vi "9229_SampleRates.vi"(9 "error in (no error)":errorcluster, 11 "Data Rate [S/s]":u32) -> (1 "error out":errorcluster, 3 "Data Rate":T1=4 items=["51.200 kS/s (NI 9229)"=1, "25.600 kS/s (NI 9229)"=2, "17.067 kS/s (NI 9229)"=3, "12.800 kS/s (NI 9229)"=4, "10.240 kS/s (NI 9229)"=5, "8.533 kS/s (NI 9229)"=6, "7.314 kS/s (NI 9229)"=7, "6.400 kS/s (NI 9229)"=8, "5.689 kS/s (NI 9229)"=9, "5.120 kS/s (NI 9229)"=10, "4.654 kS/s (NI 9229)"=11, "4.267 kS/s (NI 9229)"=12, "3.938 kS/s (NI 9229)"=13, "3.657 kS/s (NI 9229)"=14, "3.413 kS/s (NI 9229)"=15, "3.200 kS/s (NI 9229)"=16, "3.012 kS/s (NI 9229)"=17, "2.845 kS/s (NI 9229)"=18, "2.695 kS/s (NI 9229)"=19, "2.560 kS/s (NI 9229)"=20, "2.438 kS/s (NI 9229)"=21, "2.328 kS/s (NI 9229)"=22, "2.226 kS/s (NI 9229)"=23, "2.133 kS/s (NI 9229)"=24, "2.048 kS/s (NI 9229)"=25, "1.969 kS/s (NI 9229)"=26, "1.896 kS/s (NI 9229)"=27, "1.829 kS/s (NI 9229)"=28, "1.765 kS/s (NI 9229)"=29, "1.707 kS/s (NI 9229)"=30, "1.652 kS/s (NI 9229)"=31])   [LabVIEW 2017]
uses:
  <vilib>/LabVIEW Targets/FPGA/cRIO/shared/nicrio_ModuleControls/nicrio_cRIO-9229_DataRatesRing2.ctl
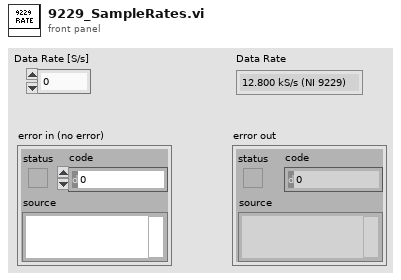
[diagram p1: front panel]
types:
  T1 = typedef "nicrio_cRIO-9229_DataRatesRing2.ctl" = u8
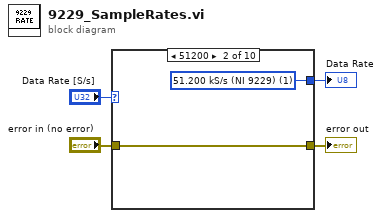
[diagram p0: block diagram]
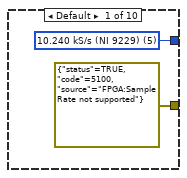
[diagram p2: hidden frame]
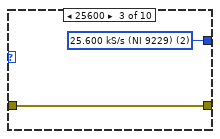
[diagram p3: hidden frame]
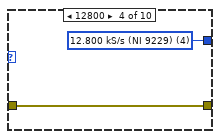
[diagram p4: hidden frame]
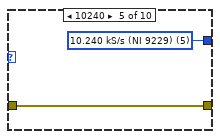
[diagram p5: hidden frame]
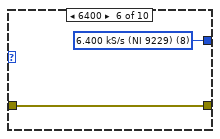
[diagram p6: hidden frame]
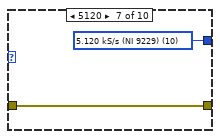
[diagram p7: hidden frame]
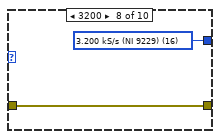
[diagram p8: hidden frame]
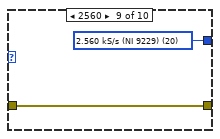
[diagram p9: hidden frame]
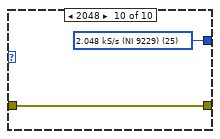
[diagram p10: hidden frame]
diagram:
  n1 = case shown="51200" "Data Rate [S/s]" {
    tunnel: [w5 w7 w9 w11 w13 w15 w17 w19 w21 w23] -> w3
    tunnel: "error in (no error)" -> [_ w8 w10 w12 w14 w16 w18 w20 w22 w24]
    tunnel: [errorcluster {"status"=TRUE, "code"=5100, "source"="FPGA:Sample Rate not supported"} ("error IO") w8 w10 w12 w14 w16 w18 w20 w22 w24] -> w1
    frame Default {
      w5 = T1 5 items=["51.200 kS/s (NI 9229)"=1, "25.600 kS/s (NI 9229)"=2, "17.067 kS/s (NI 9229)"=3, "12.800 kS/s (NI 9229)"=4, "10.240 kS/s (NI 9229)"=5, "8.533 kS/s (NI 9229)"=6, "7.314 kS/s (NI 9229)"=7, "6.400 kS/s (NI 9229)"=8, "5.689 kS/s (NI 9229)"=9, "5.120 kS/s (NI 9229)"=10, "4.654 kS/s (NI 9229)"=11, "4.267 kS/s (NI 9229)"=12, "3.938 kS/s (NI 9229)"=13, "3.657 kS/s (NI 9229)"=14, "3.413 kS/s (NI 9229)"=15, "3.200 kS/s (NI 9229)"=16, "3.012 kS/s (NI 9229)"=17, "2.845 kS/s (NI 9229)"=18, "2.695 kS/s (NI 9229)"=19, "2.560 kS/s (NI 9229)"=20, "2.438 kS/s (NI 9229)"=21, "2.328 kS/s (NI 9229)"=22, "2.226 kS/s (NI 9229)"=23, "2.133 kS/s (NI 9229)"=24, "2.048 kS/s (NI 9229)"=25, "1.969 kS/s (NI 9229)"=26, "1.896 kS/s (NI 9229)"=27, "1.829 kS/s (NI 9229)"=28, "1.765 kS/s (NI 9229)"=29, "1.707 kS/s (NI 9229)"=30, "1.652 kS/s (NI 9229)"=31] ("Data Rate")
    }
    frame 51200 {
      w7 = T1 1 items=["51.200 kS/s (NI 9229)"=1, "25.600 kS/s (NI 9229)"=2, "17.067 kS/s (NI 9229)"=3, "12.800 kS/s (NI 9229)"=4, "10.240 kS/s (NI 9229)"=5, "8.533 kS/s (NI 9229)"=6, "7.314 kS/s (NI 9229)"=7, "6.400 kS/s (NI 9229)"=8, "5.689 kS/s (NI 9229)"=9, "5.120 kS/s (NI 9229)"=10, "4.654 kS/s (NI 9229)"=11, "4.267 kS/s (NI 9229)"=12, "3.938 kS/s (NI 9229)"=13, "3.657 kS/s (NI 9229)"=14, "3.413 kS/s (NI 9229)"=15, "3.200 kS/s (NI 9229)"=16, "3.012 kS/s (NI 9229)"=17, "2.845 kS/s (NI 9229)"=18, "2.695 kS/s (NI 9229)"=19, "2.560 kS/s (NI 9229)"=20, "2.438 kS/s (NI 9229)"=21, "2.328 kS/s (NI 9229)"=22, "2.226 kS/s (NI 9229)"=23, "2.133 kS/s (NI 9229)"=24, "2.048 kS/s (NI 9229)"=25, "1.969 kS/s (NI 9229)"=26, "1.896 kS/s (NI 9229)"=27, "1.829 kS/s (NI 9229)"=28, "1.765 kS/s (NI 9229)"=29, "1.707 kS/s (NI 9229)"=30, "1.652 kS/s (NI 9229)"=31] ("Data Rate")
    }
    frame 25600 {
      w9 = T1 2 items=["51.200 kS/s (NI 9229)"=1, "25.600 kS/s (NI 9229)"=2, "17.067 kS/s (NI 9229)"=3, "12.800 kS/s (NI 9229)"=4, "10.240 kS/s (NI 9229)"=5, "8.533 kS/s (NI 9229)"=6, "7.314 kS/s (NI 9229)"=7, "6.400 kS/s (NI 9229)"=8, "5.689 kS/s (NI 9229)"=9, "5.120 kS/s (NI 9229)"=10, "4.654 kS/s (NI 9229)"=11, "4.267 kS/s (NI 9229)"=12, "3.938 kS/s (NI 9229)"=13, "3.657 kS/s (NI 9229)"=14, "3.413 kS/s (NI 9229)"=15, "3.200 kS/s (NI 9229)"=16, "3.012 kS/s (NI 9229)"=17, "2.845 kS/s (NI 9229)"=18, "2.695 kS/s (NI 9229)"=19, "2.560 kS/s (NI 9229)"=20, "2.438 kS/s (NI 9229)"=21, "2.328 kS/s (NI 9229)"=22, "2.226 kS/s (NI 9229)"=23, "2.133 kS/s (NI 9229)"=24, "2.048 kS/s (NI 9229)"=25, "1.969 kS/s (NI 9229)"=26, "1.896 kS/s (NI 9229)"=27, "1.829 kS/s (NI 9229)"=28, "1.765 kS/s (NI 9229)"=29, "1.707 kS/s (NI 9229)"=30, "1.652 kS/s (NI 9229)"=31] ("Data Rate")
    }
    frame 12800 {
      w11 = T1 4 items=["51.200 kS/s (NI 9229)"=1, "25.600 kS/s (NI 9229)"=2, "17.067 kS/s (NI 9229)"=3, "12.800 kS/s (NI 9229)"=4, "10.240 kS/s (NI 9229)"=5, "8.533 kS/s (NI 9229)"=6, "7.314 kS/s (NI 9229)"=7, "6.400 kS/s (NI 9229)"=8, "5.689 kS/s (NI 9229)"=9, "5.120 kS/s (NI 9229)"=10, "4.654 kS/s (NI 9229)"=11, "4.267 kS/s (NI 9229)"=12, "3.938 kS/s (NI 9229)"=13, "3.657 kS/s (NI 9229)"=14, "3.413 kS/s (NI 9229)"=15, "3.200 kS/s (NI 9229)"=16, "3.012 kS/s (NI 9229)"=17, "2.845 kS/s (NI 9229)"=18, "2.695 kS/s (NI 9229)"=19, "2.560 kS/s (NI 9229)"=20, "2.438 kS/s (NI 9229)"=21, "2.328 kS/s (NI 9229)"=22, "2.226 kS/s (NI 9229)"=23, "2.133 kS/s (NI 9229)"=24, "2.048 kS/s (NI 9229)"=25, "1.969 kS/s (NI 9229)"=26, "1.896 kS/s (NI 9229)"=27, "1.829 kS/s (NI 9229)"=28, "1.765 kS/s (NI 9229)"=29, "1.707 kS/s (NI 9229)"=30, "1.652 kS/s (NI 9229)"=31] ("Data Rate")
    }
    frame 10240 {
      w13 = T1 5 items=["51.200 kS/s (NI 9229)"=1, "25.600 kS/s (NI 9229)"=2, "17.067 kS/s (NI 9229)"=3, "12.800 kS/s (NI 9229)"=4, "10.240 kS/s (NI 9229)"=5, "8.533 kS/s (NI 9229)"=6, "7.314 kS/s (NI 9229)"=7, "6.400 kS/s (NI 9229)"=8, "5.689 kS/s (NI 9229)"=9, "5.120 kS/s (NI 9229)"=10, "4.654 kS/s (NI 9229)"=11, "4.267 kS/s (NI 9229)"=12, "3.938 kS/s (NI 9229)"=13, "3.657 kS/s (NI 9229)"=14, "3.413 kS/s (NI 9229)"=15, "3.200 kS/s (NI 9229)"=16, "3.012 kS/s (NI 9229)"=17, "2.845 kS/s (NI 9229)"=18, "2.695 kS/s (NI 9229)"=19, "2.560 kS/s (NI 9229)"=20, "2.438 kS/s (NI 9229)"=21, "2.328 kS/s (NI 9229)"=22, "2.226 kS/s (NI 9229)"=23, "2.133 kS/s (NI 9229)"=24, "2.048 kS/s (NI 9229)"=25, "1.969 kS/s (NI 9229)"=26, "1.896 kS/s (NI 9229)"=27, "1.829 kS/s (NI 9229)"=28, "1.765 kS/s (NI 9229)"=29, "1.707 kS/s (NI 9229)"=30, "1.652 kS/s (NI 9229)"=31] ("Data Rate")
    }
    frame 6400 {
      w15 = T1 8 items=["51.200 kS/s (NI 9229)"=1, "25.600 kS/s (NI 9229)"=2, "17.067 kS/s (NI 9229)"=3, "12.800 kS/s (NI 9229)"=4, "10.240 kS/s (NI 9229)"=5, "8.533 kS/s (NI 9229)"=6, "7.314 kS/s (NI 9229)"=7, "6.400 kS/s (NI 9229)"=8, "5.689 kS/s (NI 9229)"=9, "5.120 kS/s (NI 9229)"=10, "4.654 kS/s (NI 9229)"=11, "4.267 kS/s (NI 9229)"=12, "3.938 kS/s (NI 9229)"=13, "3.657 kS/s (NI 9229)"=14, "3.413 kS/s (NI 9229)"=15, "3.200 kS/s (NI 9229)"=16, "3.012 kS/s (NI 9229)"=17, "2.845 kS/s (NI 9229)"=18, "2.695 kS/s (NI 9229)"=19, "2.560 kS/s (NI 9229)"=20, "2.438 kS/s (NI 9229)"=21, "2.328 kS/s (NI 9229)"=22, "2.226 kS/s (NI 9229)"=23, "2.133 kS/s (NI 9229)"=24, "2.048 kS/s (NI 9229)"=25, "1.969 kS/s (NI 9229)"=26, "1.896 kS/s (NI 9229)"=27, "1.829 kS/s (NI 9229)"=28, "1.765 kS/s (NI 9229)"=29, "1.707 kS/s (NI 9229)"=30, "1.652 kS/s (NI 9229)"=31] ("Data Rate")
    }
    frame 5120 {
      w17 = T1 10 items=["51.200 kS/s (NI 9229)"=1, "25.600 kS/s (NI 9229)"=2, "17.067 kS/s (NI 9229)"=3, "12.800 kS/s (NI 9229)"=4, "10.240 kS/s (NI 9229)"=5, "8.533 kS/s (NI 9229)"=6, "7.314 kS/s (NI 9229)"=7, "6.400 kS/s (NI 9229)"=8, "5.689 kS/s (NI 9229)"=9, "5.120 kS/s (NI 9229)"=10, "4.654 kS/s (NI 9229)"=11, "4.267 kS/s (NI 9229)"=12, "3.938 kS/s (NI 9229)"=13, "3.657 kS/s (NI 9229)"=14, "3.413 kS/s (NI 9229)"=15, "3.200 kS/s (NI 9229)"=16, "3.012 kS/s (NI 9229)"=17, "2.845 kS/s (NI 9229)"=18, "2.695 kS/s (NI 9229)"=19, "2.560 kS/s (NI 9229)"=20, "2.438 kS/s (NI 9229)"=21, "2.328 kS/s (NI 9229)"=22, "2.226 kS/s (NI 9229)"=23, "2.133 kS/s (NI 9229)"=24, "2.048 kS/s (NI 9229)"=25, "1.969 kS/s (NI 9229)"=26, "1.896 kS/s (NI 9229)"=27, "1.829 kS/s (NI 9229)"=28, "1.765 kS/s (NI 9229)"=29, "1.707 kS/s (NI 9229)"=30, "1.652 kS/s (NI 9229)"=31] ("Data Rate")
    }
    frame 3200 {
      w19 = T1 16 items=["51.200 kS/s (NI 9229)"=1, "25.600 kS/s (NI 9229)"=2, "17.067 kS/s (NI 9229)"=3, "12.800 kS/s (NI 9229)"=4, "10.240 kS/s (NI 9229)"=5, "8.533 kS/s (NI 9229)"=6, "7.314 kS/s (NI 9229)"=7, "6.400 kS/s (NI 9229)"=8, "5.689 kS/s (NI 9229)"=9, "5.120 kS/s (NI 9229)"=10, "4.654 kS/s (NI 9229)"=11, "4.267 kS/s (NI 9229)"=12, "3.938 kS/s (NI 9229)"=13, "3.657 kS/s (NI 9229)"=14, "3.413 kS/s (NI 9229)"=15, "3.200 kS/s (NI 9229)"=16, "3.012 kS/s (NI 9229)"=17, "2.845 kS/s (NI 9229)"=18, "2.695 kS/s (NI 9229)"=19, "2.560 kS/s (NI 9229)"=20, "2.438 kS/s (NI 9229)"=21, "2.328 kS/s (NI 9229)"=22, "2.226 kS/s (NI 9229)"=23, "2.133 kS/s (NI 9229)"=24, "2.048 kS/s (NI 9229)"=25, "1.969 kS/s (NI 9229)"=26, "1.896 kS/s (NI 9229)"=27, "1.829 kS/s (NI 9229)"=28, "1.765 kS/s (NI 9229)"=29, "1.707 kS/s (NI 9229)"=30, "1.652 kS/s (NI 9229)"=31] ("Data Rate")
    }
    frame 2560 {
      w21 = T1 20 items=["51.200 kS/s (NI 9229)"=1, "25.600 kS/s (NI 9229)"=2, "17.067 kS/s (NI 9229)"=3, "12.800 kS/s (NI 9229)"=4, "10.240 kS/s (NI 9229)"=5, "8.533 kS/s (NI 9229)"=6, "7.314 kS/s (NI 9229)"=7, "6.400 kS/s (NI 9229)"=8, "5.689 kS/s (NI 9229)"=9, "5.120 kS/s (NI 9229)"=10, "4.654 kS/s (NI 9229)"=11, "4.267 kS/s (NI 9229)"=12, "3.938 kS/s (NI 9229)"=13, "3.657 kS/s (NI 9229)"=14, "3.413 kS/s (NI 9229)"=15, "3.200 kS/s (NI 9229)"=16, "3.012 kS/s (NI 9229)"=17, "2.845 kS/s (NI 9229)"=18, "2.695 kS/s (NI 9229)"=19, "2.560 kS/s (NI 9229)"=20, "2.438 kS/s (NI 9229)"=21, "2.328 kS/s (NI 9229)"=22, "2.226 kS/s (NI 9229)"=23, "2.133 kS/s (NI 9229)"=24, "2.048 kS/s (NI 9229)"=25, "1.969 kS/s (NI 9229)"=26, "1.896 kS/s (NI 9229)"=27, "1.829 kS/s (NI 9229)"=28, "1.765 kS/s (NI 9229)"=29, "1.707 kS/s (NI 9229)"=30, "1.652 kS/s (NI 9229)"=31] ("Data Rate")
    }
    frame 2048 {
      w23 = T1 25 items=["51.200 kS/s (NI 9229)"=1, "25.600 kS/s (NI 9229)"=2, "17.067 kS/s (NI 9229)"=3, "12.800 kS/s (NI 9229)"=4, "10.240 kS/s (NI 9229)"=5, "8.533 kS/s (NI 9229)"=6, "7.314 kS/s (NI 9229)"=7, "6.400 kS/s (NI 9229)"=8, "5.689 kS/s (NI 9229)"=9, "5.120 kS/s (NI 9229)"=10, "4.654 kS/s (NI 9229)"=11, "4.267 kS/s (NI 9229)"=12, "3.938 kS/s (NI 9229)"=13, "3.657 kS/s (NI 9229)"=14, "3.413 kS/s (NI 9229)"=15, "3.200 kS/s (NI 9229)"=16, "3.012 kS/s (NI 9229)"=17, "2.845 kS/s (NI 9229)"=18, "2.695 kS/s (NI 9229)"=19, "2.560 kS/s (NI 9229)"=20, "2.438 kS/s (NI 9229)"=21, "2.328 kS/s (NI 9229)"=22, "2.226 kS/s (NI 9229)"=23, "2.133 kS/s (NI 9229)"=24, "2.048 kS/s (NI 9229)"=25, "1.969 kS/s (NI 9229)"=26, "1.896 kS/s (NI 9229)"=27, "1.829 kS/s (NI 9229)"=28, "1.765 kS/s (NI 9229)"=29, "1.707 kS/s (NI 9229)"=30, "1.652 kS/s (NI 9229)"=31] ("Data Rate")
    }
  }
  "Data Rate" <- w3
  "error out" <- w1
